vi "Create ToolStripLabel.vi"(8 "error in (no error)":errorcluster caption="错误输入（无错误）", 11 "text":string) -> (0 "error out":errorcluster caption="错误输出", 3 "ToolStripLabel 输出":refnum<class "ToolStripLabel.lvclass"> caption="DNL_LabVIEW Object out")   [LabVIEW 2013, in "ToolStripLabel.lvclass"]
uses:
  ToolStripLabel.lvclass
  System.Windows.Forms
  ToolStripLabel.lvclass/ToolStripLabel.ctl
panel:
  in  "ToolStripLabel 输入":refnum<class "ToolStripLabel.lvclass"> caption="DNL_LabVIEW Object in"
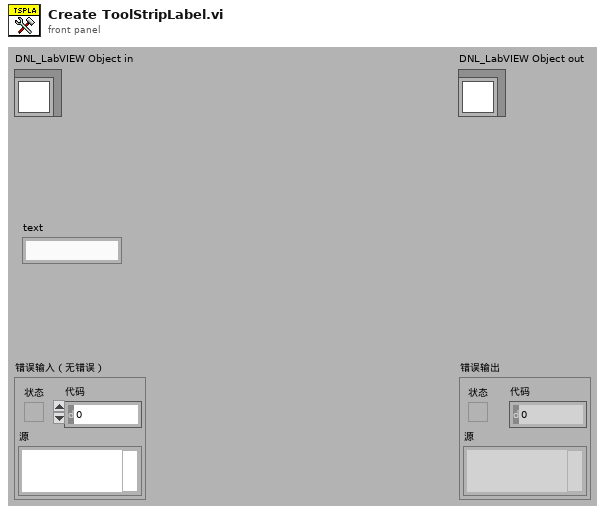
[diagram p1: front panel]
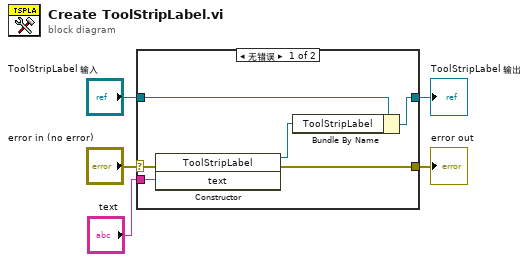
[diagram p0: block diagram]
diagram:
  n1 = case shown="无错误" "error in (no error)" {
    selector: "error in (no error)" -> [w7 w13]
    tunnel: [w6 w13] -> w4
    tunnel: [w9 w12] -> w2
    tunnel: "ToolStripLabel 输入" -> [w10 w12]
    tunnel: "text" -> [w11 _]
    frame No Error {
      n2 = constructor class="ToolStripLabel"(error in=w7, "text"=w11) -> (reference out=w8:refnum<k24>, error out=w6:errorcluster)  [unwired: 2 in, 2 out]
      n3 = Bundle By Name(cluster=w10, "ToolStripLabel"=w8) -> (w9:refnum<class "ToolStripLabel.lvclass">)
    }
    frame Error {
    }
  }
  "error out" <- w4
  "ToolStripLabel 输出" <- w2
